vi "Picolog Temperature to Waveform.vi"(8 "Error In":errorcluster, 9 "Temperature":dbl[](array[numeric])) -> (0 "Error Out":errorcluster, 1 "Temperature Waveform":waveform(dbl)[](array[waveform]), 2 "Sample Interval [s]":dbl format="%#_2g")   [LabVIEW 2016]
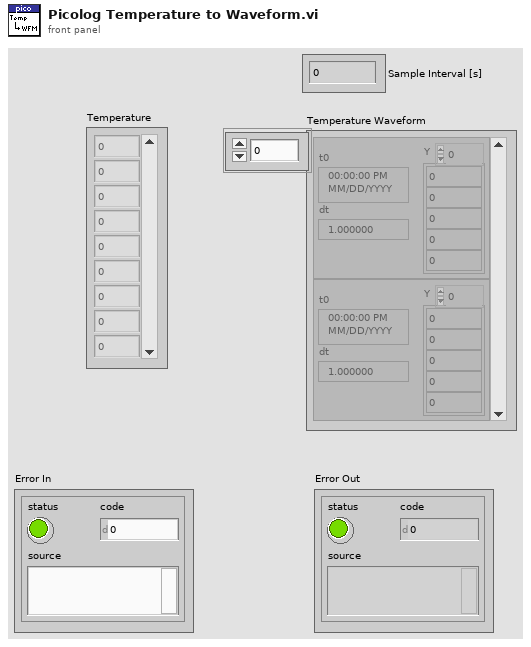
[diagram p1: front panel]
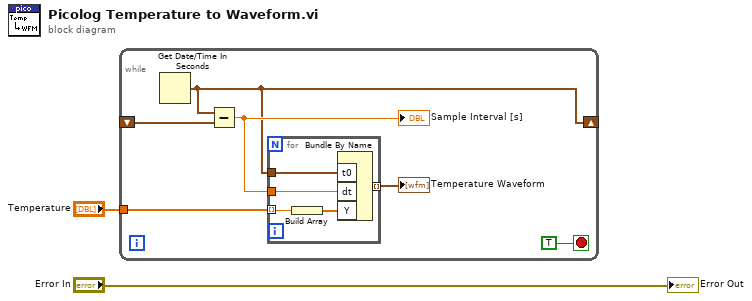
[diagram p0: block diagram]
diagram:
  n1 = while {
    tunnel: "Temperature" -> [w5]
    shift-right: [w4] -> _
    shift-left: _ -> [w8]
    stop <- TRUE stop-if-true
    n2 = Get Date/Time In Seconds() -> (seconds since 1Jan1904=w4:timestamp)
    n3 = Subtract(x=w4, y=w8) -> (x-y=w7:dbl)
    "Sample Interval [s]" <- w7
    n4 = for {
      tunnel: w5 -> [w13] mode=indexing
      tunnel: [w12] -> w6 mode=indexing
      tunnel: w4 -> [w11]
      tunnel: w7 -> [w10]
      n5 = Build Array(w13) -> (w9:dbl[])
      n6 = Bundle By Name("t0"=w11, "dt"=w10, "Y"=w9) -> (w12:waveform(dbl))  [unwired: 1 in]
    }
    "Temperature Waveform" <- w6
  }
  "Error Out" <- "Error In"
